vi "test Deployment SLSC Switch and RaF CD.vi"(8 "error in (no error)":errorcluster, 11 "TestCase in":refnum<class "SLSC Switch System Tests.lvclass">) -> (0 "error out":errorcluster, 3 "TestCase out":refnum<class "SLSC Switch System Tests.lvclass">)   [LabVIEW 2017, in "SLSC Switch System Tests.lvclass"]
uses:
  SLSC Switch System Tests.lvclass
  <vilib>/addons/_JKI Toolkits/VI Tester/TestCase.llb/TestCase.lvclass
  C:/Program Files (x86)/National Instruments/LabVIEW 2017/vi.lib/addons/_JKI Toolkits/VI Tester/TestCase.llb/TestCase.lvclass
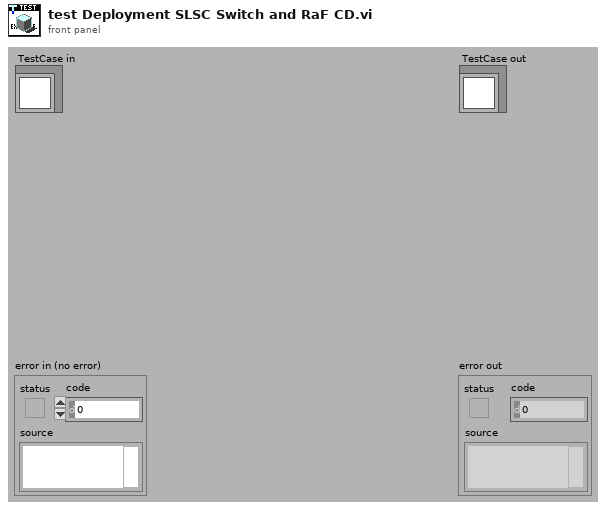
[diagram p1: front panel]
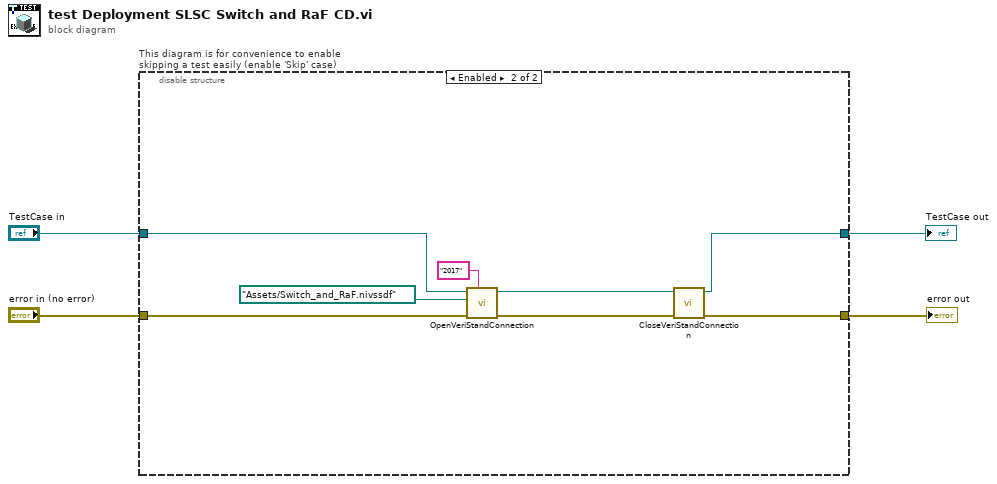
[diagram p0: block diagram]
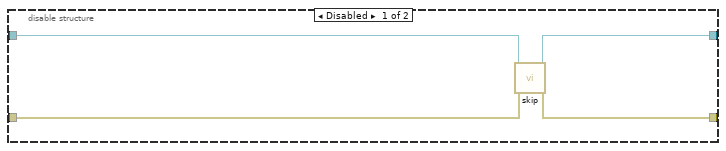
[diagram p2: hidden frame]
diagram:
  n1 = disable-structure "This diagram is for convenience to enable skipping a test easily (enable 'Skip' case)" shown="Enabled" {
    disable-tunnel: "TestCase in" -> [w8 w16]
    disable-tunnel: [w7 w14] -> w1
    disable-tunnel: [w6 w13] -> w3
    disable-tunnel: "error in (no error)" -> [w5 w15]
    frame Disabled {
      n2 = call <vilib>:"skip.vi"("error in (no error)"=w5, "TestCase in"=w8) -> ("error out"=w6:errorcluster, "TestCase out"=w7:refnum<class "SLSC Switch System Tests.lvclass">)  [unwired: 8 in]
    }
    frame Enabled {
      n3 = call-dynamic "OpenVeriStandConnection.vi"("Minimum VeriStand Version (2016)"="2017" ("Minimum VeriStand Version (2015)"), "error in (no error)"=w15, "System Definition File"=path "Assets/Switch_and_RaF.nivssdf", "VeriStand Test Case in"=w16) -> ("error out"=w9:errorcluster, "VeriStand Test Case out"=w10:refnum<class "SLSC Switch System Tests.lvclass">)  [unwired: 5 in, 1 out]
      n4 = call-dynamic "CloseVeriStandConnection.vi"("error in (no error)"=w9, "VeriStand Test Case in"=w10) -> ("error out"=w13:errorcluster, "VeriStand Test Case out"=w14:refnum<class "SLSC Switch System Tests.lvclass">)  [unwired: 8 in]
    }
  }
  "error out" <- w3
  "TestCase out" <- w1
